vi "Do.vi"(8 "error in (no error)":errorcluster, 10 "Actor in":refnum<class "Actor.lvclass">, 11 "Terminate Sequencer Msg":refnum<class "Terminate Sequencer Msg.lvclass">) -> (0 "error out":errorcluster, 2 "Actor out":refnum<class "Actor.lvclass">)   [LabVIEW 2020, in "Sequencer.lvlib" / "Terminate Sequencer Msg.lvclass"]
doc: "Call the Stop Msg Do method to stop the Sequencer actor."
uses:
  Terminate Sequencer Msg.lvclass
  PPL/HDH.Actor Framework.Core.Actor.lvlibp/1abvi3w/vi.lib/ActorFramework/Actor/Actor.lvclass
  PPL/HDH.Actor Framework.Core.Actor.lvlibp/1abvi3w/vi.lib/ActorFramework/Stop Msg/Stop Msg.lvclass
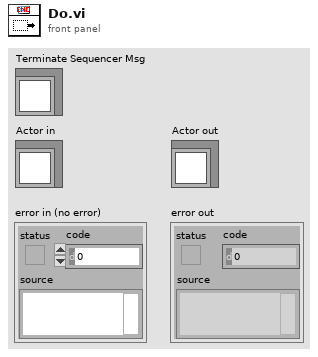
[diagram p1: front panel]
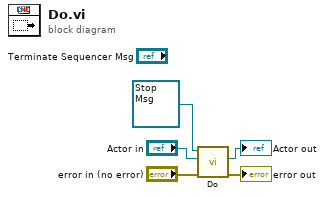
[diagram p0: block diagram]
diagram:
  n1 = call-dynamic "Do.vi"("error in (no error)"="error in (no error)", "Actor in"="Actor in", "Stop Msg"=refnum<class "Stop Msg.lvclass"> refnum ("Actor Framework:Stop Msg")) -> ("error out"=→"error out":errorcluster, "Actor out"=→"Actor out":refnum<class "Actor.lvclass">)  [unwired: 7 in]
